vi "Warp Affine (ARGB).vi"(4 "Border Colour (Default: Black)":T2={"Alpha"=255, "RGB"=0}, 5 "Boarder Type (Default: DEFAULT)":T3=enum."DEFAULT", 6 "Required Destination Size":T6, 7 "Interpolation Mode (Default: CUBIC)":T5=enum."CUBIC", 8 "error in (no error)":errorcluster, 9 "2x3 Affine Matrix":T1, 10 "ARGB Destination Image in":T4, 11 "ARGB Source Image in":T4) -> (0 "error out":errorcluster, 3 "ARGB  Destination Image":T4)   [LabVIEW 2020, in "image.lvlib"]
doc: "Warp the Source Image according to the given 2x3 Affine Matrix."
uses:
  image.lvlib
  ARGB Image.ctl
  common/Image Size (Integer).ctl
  Interpolation Mode.ctl
  Border Type.ctl
  ARGB Colour.ctl
  <vilib>/Analysis/Matrix/Datatypes/RealMatrix.ctl
  b7e6b07f-7daf-4958-9fc0-179f1836a141.vi
  b7e6b07f-7daf-4958-9fc0-179f1836a141.vi/0c263cf4-9042-4d44-b92e-dafa676e1650.vi
  <vilib>/Utility/error.llb/Error Cluster From Error Code.vi
  common/common.lvlib
  <vilib>/Analysis/Matrix/NI_Matrix.lvlib
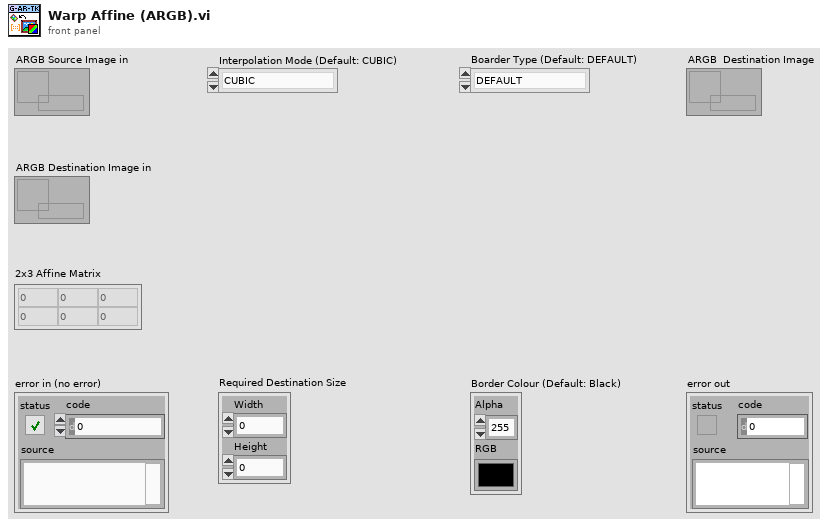
[diagram p1: front panel]
types:
  T1 = typedef "NI_Matrix.lvlib/RealMatrix.ctl" = dbl[][]
  T2 = typedef "image.lvlib/ARGB Colour.ctl" = cluster{"Alpha":u8, "RGB":u32}
  T3 = typedef "image.lvlib/Border Type.ctl" = enum8{"CONSTANT", "REPLICATE", "REFLECT", "WRAP", "TRANSPARENT", "DEFAULT", "ISOLATED"}
  T4 = typedef "image.lvlib/ARGB Image.ctl" = refnum<data-value>
  T5 = typedef "image.lvlib/Interpolation Mode.ctl" = enum8{"NEAREST", "LINEAR", "CUBIC", "AREA", "LANCZOS", "LINEAR_EXACT", "NEAREST_EXACT", "MAX"}
  T6 = typedef "common.lvlib/Image Size (Integer).ctl" = cluster{"Width":u16, "Height":u16}
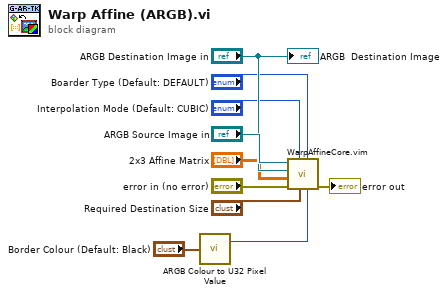
[diagram p0: block diagram]
diagram:
  n1 = call "ARGB Colour to U32 Pixel Value.vi"("ARGB Colour"="Border Colour (Default: Black)") -> ("U32 Colour"=w1:u32)
  n2 = call "WarpAffineCore.vim"("Border Colour"=w1, "Boarder Type"="Boarder Type (Default: DEFAULT)", "Destination Size"="Required Destination Size", "Interpolation Mode"="Interpolation Mode (Default: CUBIC)", "error in (no error)"="error in (no error)", "Affine"="2x3 Affine Matrix", "Dst"="ARGB Destination Image in", "Src"="ARGB Source Image in") -> ("error out"=→"error out":errorcluster)  [unwired: 3 in]
  "ARGB  Destination Image" <- "ARGB Destination Image in"
